vi "DemoReadDigital.vi"() -> ()   [LabVIEW 2009]
uses:
  <vilib>/NXT/Block Support/NXT_InputPort.ctl
  <vilib>/NXT/Dual Mode Library/Waits/Wait_Num(msec).vi
  <vilib>/NXT/Dual Mode Library/Display/drawText.vi
panel:
  in  "stop":bool
  # "Demo Digital Read"
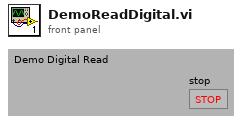
[diagram p1: front panel]
types:
  T1 = typedef "NXT_InputPort.ctl" = u8
  T2 = typedef "LVHSConnector.ctl" = cluster{"error":errorcluster, "address":string, "NXT #":i32, "Show Error":bool, "Connection":u16}
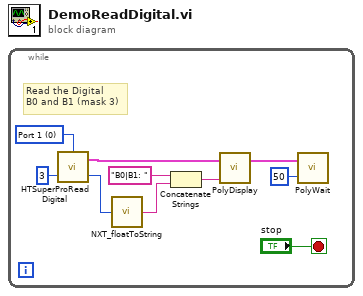
[diagram p0: block diagram]
diagram:
  n1 = while {
    stop <- "stop" stop-if-true
    w1 = T1 0 items=["Port 1", "Port 2", "Port 3", "Port 4"] ("Port")
    # "Read the Digital \nB0 and B1 (mask 3)"
    n2 = call "HTSuperProReadDigital.vi"("Mask"=u8 3, "Port"=w1) -> ("Digital Value"=w3:u8, "NXT"=w4:T2)  [unwired: 2 in]
    n3 = call <vilib>:"NXT_floatToString.vi"("number"=w3) -> ("string"=w7:string)
    n4 = Concatenate Strings("B0|B1: " ("string"), w7) -> (w9:string)
    n5 = call-poly <vilib>:"PolyDisplay.vi"("Text"=w9, "NXT"=w4) -> ("NXT"=w5:T2)  [unwired: 2 in]
    n6 = call-poly <vilib>:"PolyWait.vi"("Time (100 msec)"=u32 50, "NXT"=w5) -> ()  [unwired: 2 in, 1 out]
  }
